vi "Convert to hex string.vi"(11 "Trace in":string[][](table)=[["", "", "", "", ""], ["", "", "", "", ""], ["", "", "", "", ""], ["", "", "", "", ""], ["", "", "", "", ""], ["", "", "", "", ""]]) -> (3 "Trace out":string[][](table))   [LabVIEW 2025, in "CAN-LIN Raw Bus Capture UI.lvlib"]
uses:
  CAN-LIN Raw Bus Capture UI.lvlib
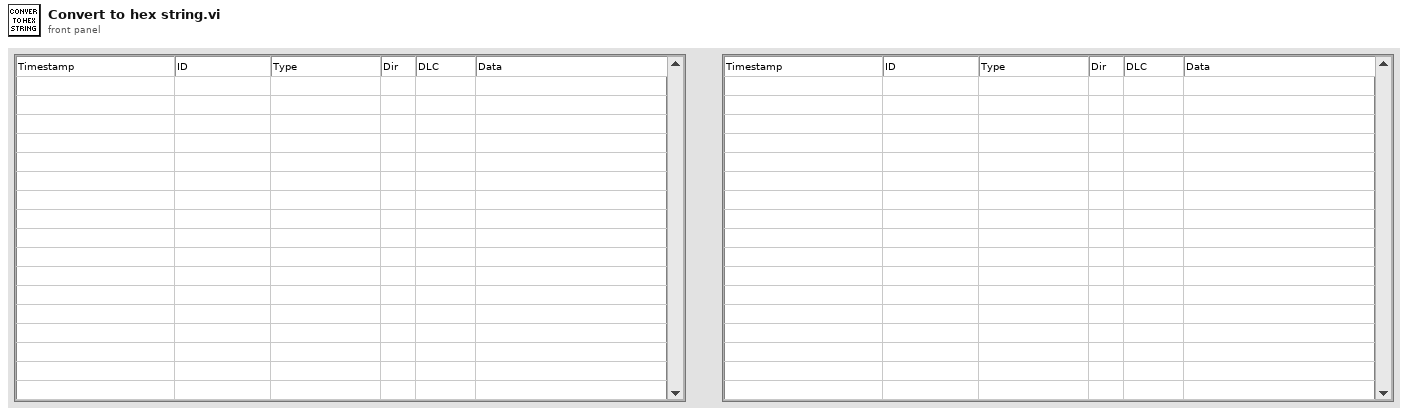
[diagram p1: front panel]
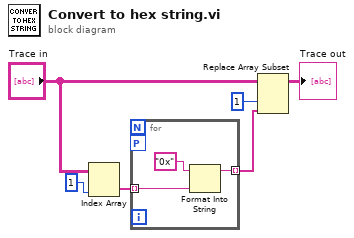
[diagram p0: block diagram]
diagram:
  n1 = Index Array(array="Trace in", index (col)=1 ("disabled index (col)")) -> (element=w4:string[])  [unwired: 1 in]
  n2 = for {
    tunnel: w4 -> [w9] mode=indexing
    workers-P: _ -> [_]
    tunnel: [w8] -> w1 mode=indexing
    n3 = Format Into String(initial string="0x", w9) -> (resulting string=w8:string)  [unwired: 2 in, 1 out]
  }
  n4 = Replace Array Subset(array="Trace in", new element=w1, index (col)=1 ("disabled index (col)")) -> (→"Trace out":string[][])  [unwired: 1 in]
